vi "1L14_DSA_per_txt-de-xi.vi"(1 "xi":dbl[](array[numeric])) -> (0 "Période":string[](array[string]))   [LabVIEW 2010, in "lv_01.lvlib"]
uses:
  lv_01.lvlib
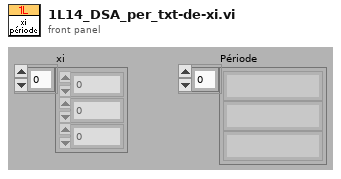
[diagram p1: front panel]
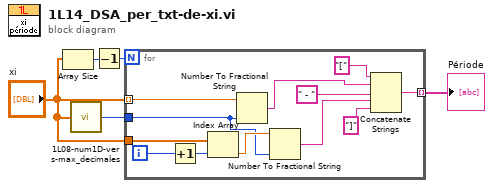
[diagram p0: block diagram]
diagram:
  n1 = Array Size(array="xi") -> (size(s)=w4:i32)
  n2 = call "1L08-num1D-vers-max_decimales.vi"("num. déc. (1D)"="xi") -> ("Max déc."=w2:i32)
  n3 = Decrement(x=w4) -> (x-1=w5:i32)
  n4 = for {
    N: w5 -> [_]
    tunnel: "xi" -> [w15]
    tunnel: "xi" -> [w13] mode=indexing
    tunnel: [w7] -> w1 mode=indexing
    tunnel: w2 -> [w6]
    i -> [w16]
    n5 = Increment(x=w16) -> (x+1=w17:i32)
    n6 = Index Array(array=w15, index=w17) -> (element=w14:dbl)
    n7 = Number To Fractional String(number=w13, precision (6)=w6) -> (F-format string=w11:string)  [unwired: 2 in]
    n8 = Number To Fractional String(number=w14, precision (6)=w6) -> (F-format string=w9:string)  [unwired: 2 in]
    n9 = Concatenate Strings("[" ("chaîne"), w11, " - " ("chaîne"), w9, "]" ("chaîne")) -> (w7:string)
  }
  "Période" <- w1
